vi "Autonomous Independent.vi"() -> ()   [LabVIEW 2020]
doc: "This VI is called when autonomous begins, and will automatically be terminated when autonomous ends. You can carry out timed or sensor driven robot movement independently without needing to return to the caller."
uses:
  <vilib>/Rock Robotics/Network Tables/NT Read String.vi
  <vilib>/Utility/file.llb/Read Delimited Spreadsheet (DBL).vi
  Robot Global Data.vi
  <vilib>/Rock Robotics/WPI/RobotDrive/WPI_RobotDriveArcadeDrive_Standard(NoSaturation).vi
  <vilib>/Rock Robotics/Network Tables/NT Write Numeric Array.vi
panel:
  out "Current Movement, for debugging":T1 {"Y Joystick Value" scale=1.0..-1.0; "X Joystick Value" scale=-1.0..1.0}
  in  "Array of robot movements":T2(array[cluster])=[{"X Joystick Value"=0.39393939393939403, "Y Joystick Value"=0.0, "Delay (sec)"=1.0, "Movement Name"="turn"}, {"X Joystick Value"=-0.3737373737373737, "Y Joystick Value"=0.0, "Delay (sec)"=1.0, "Movement Name"="turn back"}] {"Y Joystick Value" scale=1.0..-1.0; "X Joystick Value" scale=-1.0..1.0}
  # "Be sure to right-click and choose Data Operations>>Make Current Value default if you want to save the array values with the VI"
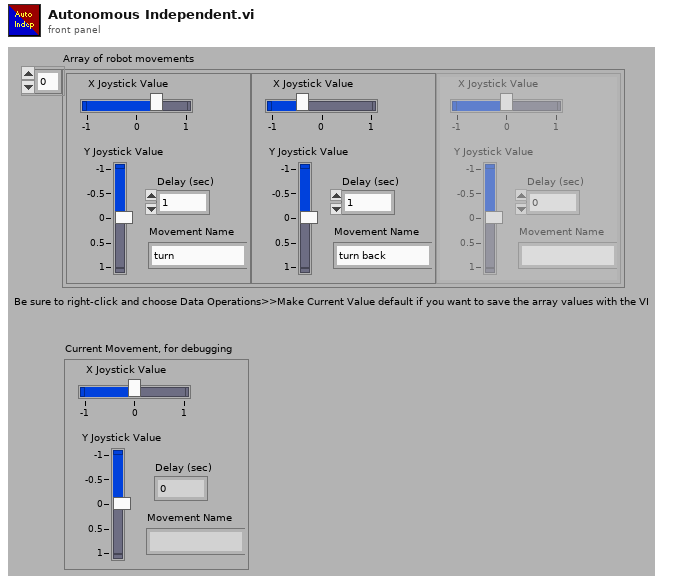
[diagram p1: front panel]
types:
  T1 = cluster{"X Joystick Value":dbl, "Y Joystick Value":dbl, "Delay (sec)":dbl, "Movement Name":string}
  T2 = cluster{"X Joystick Value":dbl, "Y Joystick Value":dbl, "Delay (sec)":dbl, "Movement Name":string}[]
  T3 = typedef "WPI_JoystickDevRef.ctl" = cluster{"Device":T4}
  T4 = typedef "WPI_JoystickDeviceEnum.ctl" = enum16{"USB 0", "USB 1", "USB 2", "USB 3", "USB 4", "USB 5"}
  T5 = typedef "WPI_RobotDriveDevRef.ctl" = cluster{"DevStatus":errorcluster, "Motors[]":T6[], "Square Inputs":bool, "Max Output":dbl}
  T6 = typedef "WPI_MotorControlDeviceRef.ctl" = cluster{"DeviceStatus":errorcluster, "Type":T7, "PWM":cluster{"PWM Channel":T8, "DeadBand":T9}, "CAN":cluster{"Device Number":u8, "SetOutput VI Ref":variant, "GetOutput VI Ref":variant, "Enable VI Ref":variant, "Disable VI Ref":variant, "Data":variant}, "Invert":bool, "DIO PWM":cluster{"PWM \"Enable\" Channel":T8, "DIOChannel":T10, "PWM Rate":dbl}}
  T7 = typedef "WPI_MotorControlType.ctl" = enum16{"PWM", "CAN", "DIO PWM"}
  T8 = typedef "FPGA_DIOPWMChannel.ctl" = enum8{"PWM 0", "PWM 1", "PWM 2", "PWM 3", "PWM 4", "PWM 5", "PWM 6", "PWM 7", "PWM 8", "PWM 9", "PWM MXP 0", "PWM MXP 1", "PWM MXP 2", "PWM MXP 3", "PWM MXP 4", "PWM MXP 5", "PWM MXP 6", "PWM MXP 7", "PWM MXP 8", "PWM MXP 9", "Invalid"}
  T9 = typedef "WPI_PWMDeadband.ctl" = cluster{"Name":string, "maxPositivePwm":i32, "minPositivePwm":i32, "centerPwm":i32, "maxNegativePwm":i32, "minNegativePwm":i32, "angularRange":u16}
  T10 = typedef "FPGA_DIOChannel.ctl" = enum8{"DIO 0", "DIO 1", "DIO 2", "DIO 3", "DIO 4", "DIO 5", "DIO 6", "DIO 7", "DIO 8", "DIO 9", "DIO MXP 0", "DIO MXP 1", "DIO MXP 2", "DIO MXP 3", "DIO MXP 4", "DIO MXP 5", "DIO MXP 6", "DIO MXP 7", "DIO MXP 8", "DIO MXP 9", "DIO MXP 10", "DIO MXP 11", "DIO MXP 12", "DIO MXP 13", "DIO MXP 14", "DIO MXP 15", "SPI Port CS1", "SPI Port CS2", "SPI Port CS3", "SPI Port MISO", "SPI Port MOSI", "Invalid"}
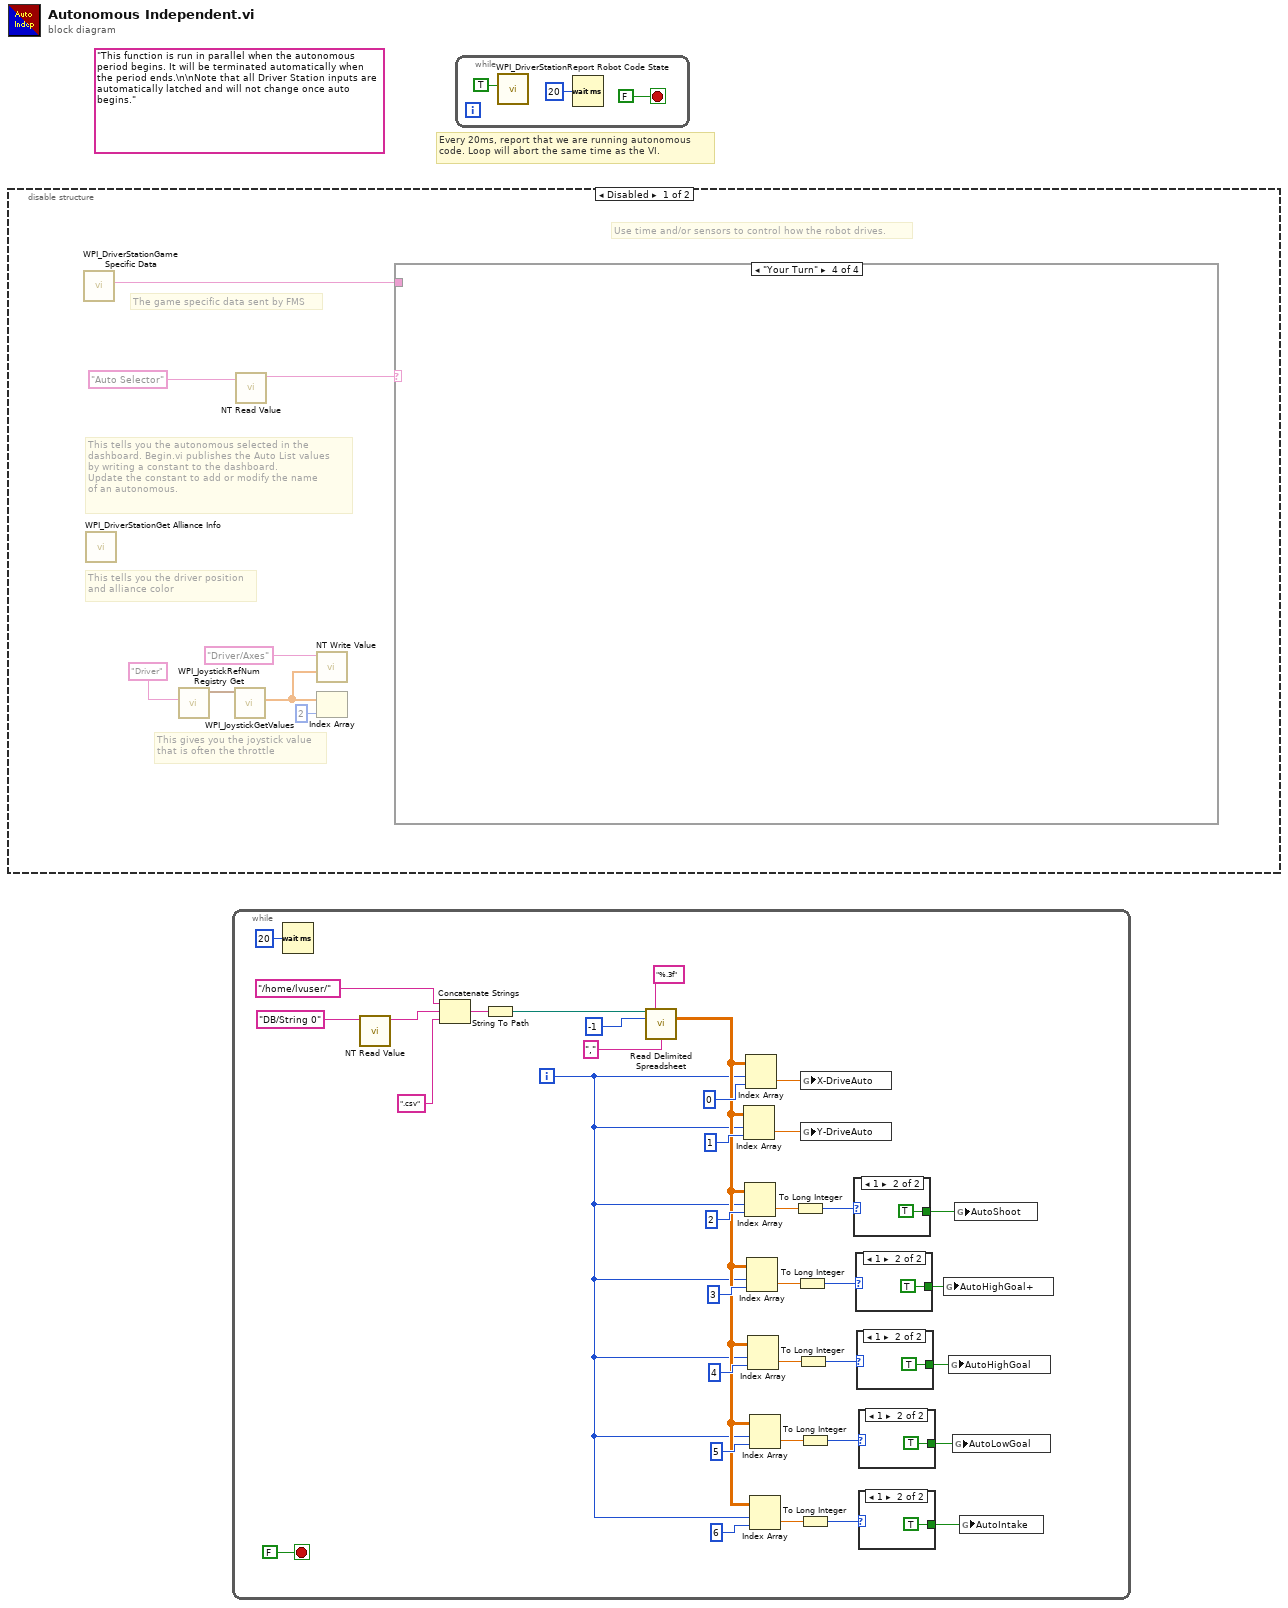
[diagram p0: block diagram]
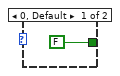
[diagram p2: hidden frame]
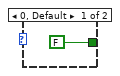
[diagram p3: hidden frame]
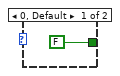
[diagram p4: hidden frame]
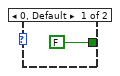
[diagram p5: hidden frame]
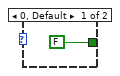
[diagram p6: hidden frame]
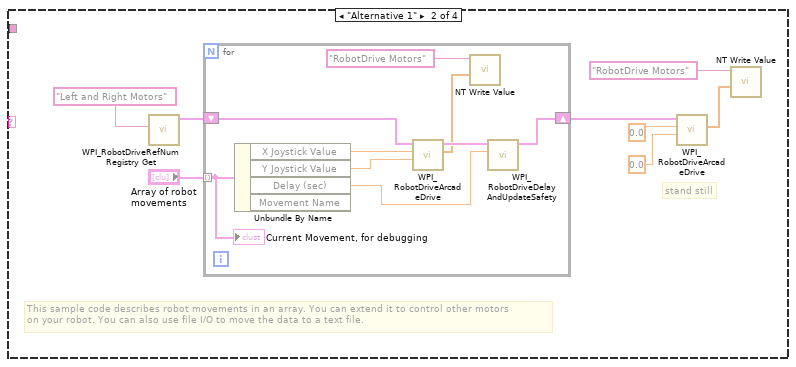
[diagram p8: hidden frame]
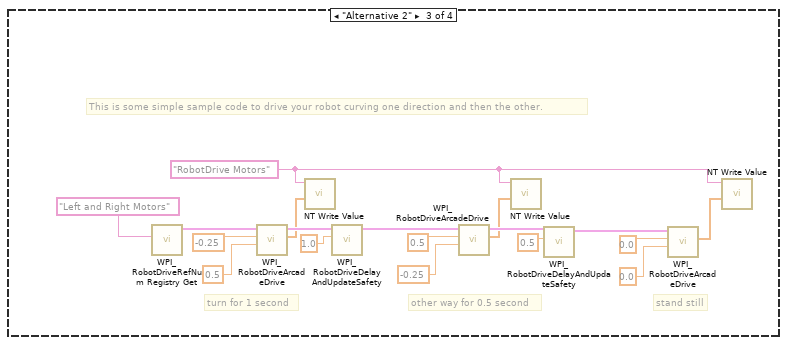
[diagram p9: hidden frame]
diagram:
  (unwired) "This function is run in parallel when the autonomous period begins. It will be terminated automatically when the period ends.\n\nNote that all Driver Station inputs are automatically latched and will not change once auto begins."
  # "Every 20ms, report that we are running autonomous\ncode. Loop will abort the same time as the VI."
  n1 = disable-structure shown="Disabled" {
    frame Disabled {
      # "This gives you the joystick value\nthat is often the throttle"
      # "The game specific data sent by FMS"
      # "This tells you the autonomous selected in the \ndashboard. Begin.vi publishes the Auto List values\nby writing a constant to the dashboard.\nUpdate the constant to add or modify the name\nof an autonomous."
      # "Use time and/or sensors to control how the robot drives."
      # "This tells you the driver position\nand alliance color"
      n2 = call <vilib>:"WPI_DriverStationGame Specific Data.vi"() -> ("Game Specific Data"=w6:string)  [unwired: 11 in]
      n3 = call <vilib>:"WPI_DriverStationGet Alliance Info.vi"() -> ()  [unwired: 12 out]
      n4 = call <vilib>:"WPI_JoystickRefNum Registry Get.vi"("refnum name"="Driver") -> ("JoystickDevRef"=w4:T3)  [unwired: 1 in, 9 out]
      n5 = call <vilib>:"WPI_JoystickGetValues.vi"("JoystickDevRef"=w4) -> ("Axes"=w2:dbl[])  [unwired: 6 in, 4 out]
      n6 = call-poly <vilib>:"NT Read Value.vi"("Name"="Auto Selector") -> ("String"=w7:string)  [unwired: 9 in, 1 out]
      n7 = call-poly <vilib>:"NT Write Value.vi"("Numeric Array"=w2, "Name"="Driver/Axes") -> ()  [unwired: 9 in, 1 out]
      n8 = Index Array(array=w2, index=2) -> ()  [unwired: 1 out]
      n9 = case shown="\"Your Turn\"" w7 {
        tunnel: w6 -> [_ _ _ _]
        frame Default {
          # "You can put your main auto here, or you can right-click on the case and make any\nother frame be the default case."
          # "This is the frame that will execute if no selection is made, or if it is not recognized"
        }
        frame "Alternative 1" {
          # "stand still"
          # "This sample code describes robot movements in an array. You can extend it to control other motors\non your robot. You can also use file I/O to move the data to a text file."
          n10 = call <vilib>:"WPI_RobotDriveRefNum Registry Get.vi"("refnum name"="Left and Right Motors") -> ("RobotDriveDevRef"=w15:T5)  [unwired: 1 in, 9 out]
          n11 = for {
            shift-right: [w23] -> w10
            shift-left: w15 -> [w24]
            tunnel: "Array of robot movements" -> [w19] mode=indexing
            n12 = Unbundle By Name(w19) -> ("X Joystick Value"=w22:dbl, "Y Joystick Value"=w21:dbl, "Delay (sec)"=w20:dbl)  [unwired: 1 out]
            n13 = call-poly <vilib>:"WPI_RobotDriveArcadeDrive.vi"("Y axis value"=w21, "X axis value"=w22, "RobotDriveDevRef"=w24) -> ("Motor Values"=w17:dbl[], "RobotDriveDevRef"=w25:T5)  [unwired: 1 in, 6 out]
            n14 = call-poly <vilib>:"NT Write Value.vi"("Numeric Array"=w17, "Name"="RobotDrive Motors") -> ()  [unwired: 9 in, 1 out]
            n15 = call <vilib>:"WPI_RobotDriveDelayAndUpdateSafety.vi"("Delay (s)"=w20, "RobotDriveDevRef"=w25) -> ("RobotDriveDevRef 2"=w23:T5)  [unwired: 8 in, 1 out]
            "Current Movement, for debugging" <- w19
          }
          n16 = call-poly <vilib>:"WPI_RobotDriveArcadeDrive.vi"("Y axis value"=0.0 ("X axis value"), "X axis value"=0.0, "RobotDriveDevRef"=w10) -> ("Motor Values"=w13:dbl[])  [unwired: 1 in, 7 out]
          n17 = call-poly <vilib>:"NT Write Value.vi"("Numeric Array"=w13, "Name"="RobotDrive Motors") -> ()  [unwired: 9 in, 1 out]
        }
        frame "Alternative 2" {
          w27 = "RobotDrive Motors" ("Name")
          # "This is some simple sample code to drive your robot curving one direction and then the other."
          # "stand still"
          # "other way for 0.5 second"
          # "turn for 1 second"
          n18 = call <vilib>:"WPI_RobotDriveRefNum Registry Get.vi"("refnum name"="Left and Right Motors") -> ("RobotDriveDevRef"=w43:T5)  [unwired: 1 in, 9 out]
          n19 = call-poly <vilib>:"WPI_RobotDriveArcadeDrive.vi"("Y axis value"=0.5 ("X axis value"), "X axis value"=-0.25, "RobotDriveDevRef"=w43) -> ("Motor Values"=w26:dbl[], "RobotDriveDevRef"=w36:T5)  [unwired: 1 in, 6 out]
          n20 = call-poly <vilib>:"NT Write Value.vi"("Numeric Array"=w26, "Name"=w27) -> ()  [unwired: 9 in, 1 out]
          n21 = call <vilib>:"WPI_RobotDriveDelayAndUpdateSafety.vi"("Delay (s)"=1.0, "RobotDriveDevRef"=w36) -> ("RobotDriveDevRef 2"=w37:T5)  [unwired: 8 in, 1 out]
          n22 = call-poly <vilib>:"WPI_RobotDriveArcadeDrive.vi"("Y axis value"=-0.25 ("X axis value"), "X axis value"=0.5, "RobotDriveDevRef"=w37) -> ("Motor Values"=w28:dbl[], "RobotDriveDevRef"=w38:T5)  [unwired: 1 in, 6 out]
          n23 = call-poly <vilib>:"NT Write Value.vi"("Numeric Array"=w28, "Name"=w27) -> ()  [unwired: 9 in, 1 out]
          n24 = call <vilib>:"WPI_RobotDriveDelayAndUpdateSafety.vi"("Delay (s)"=0.5, "RobotDriveDevRef"=w38) -> ("RobotDriveDevRef 2"=w39:T5)  [unwired: 8 in, 1 out]
          n25 = call-poly <vilib>:"WPI_RobotDriveArcadeDrive.vi"("Y axis value"=0.0 ("X axis value"), "X axis value"=0.0, "RobotDriveDevRef"=w39) -> ("Motor Values"=w29:dbl[])  [unwired: 1 in, 7 out]
          n26 = call-poly <vilib>:"NT Write Value.vi"("Numeric Array"=w29, "Name"=w27) -> ()  [unwired: 9 in, 1 out]
        }
        frame "Your Turn" {
        }
      }
    }
    frame Enabled {
    }
  }
  n27 = while {
    i -> [w50]
    stop <- FALSE stop-if-true
    n28 = Wait (ms)(milliseconds to wait=u32 20) -> ()  [unwired: 1 out]
    n29 = call-poly <vilib>:"NT Read Value.vi"("Name"="DB/String 0") -> ("String"=w47:string)  [unwired: 9 in, 1 out]
    n30 = Concatenate Strings("/home/lvuser/", w47, ".csv") -> (w45:string)
    n31 = String To Path(string=w45) -> (path=w44:path)
    n32 = call-poly <vilib>:"Read Delimited Spreadsheet.vi"("file path (dialog if empty)"=w44, "format (%.3f)"="%.3f", "number of rows (all:-1)"=-1, "delimiter (\\t)"="," ("delimiter (\\t)")) -> ("all rows"=w51:dbl[][])  [unwired: 6 in, 5 out]
    n33 = Index Array(array=w51, index (row)=w50, index (col)=1 ("disabled index (col)")) -> (element=w72:dbl)
    n34 = Index Array(array=w51, index (row)=w50, index (col)=2 ("disabled index (col)")) -> (element=w70:dbl)
    n35 = Index Array(array=w51, index (row)=w50, index (col)=0 ("disabled index (col)")) -> (element=w73:dbl)
    n36 = Index Array(array=w51, index (row)=w50, index (col)=3 ("disabled index (col)")) -> (element=w66:dbl)
    n37 = Index Array(array=w51, index (row)=w50, index (col)=4 ("disabled index (col)")) -> (element=w62:dbl)
    n38 = Index Array(array=w51, index (row)=w50, index (col)=5 ("disabled index (col)")) -> (element=w58:dbl)
    n39 = Index Array(array=w51, index (row)=w50, index (col)=6 ("disabled index (col)")) -> (element=w54:dbl)
    n40 = To Long Integer(number=w70) -> (32bit integer=w68:i32)
    n41 = To Long Integer(number=w66) -> (32bit integer=w64:i32)
    n42 = To Long Integer(number=w62) -> (32bit integer=w60:i32)
    n43 = To Long Integer(number=w58) -> (32bit integer=w56:i32)
    n44 = To Long Integer(number=w54) -> (32bit integer=w52:i32)
    n45 = global write "Robot Global Data.vi" "X-DriveAuto"(w73) -> ()
    n46 = global write "Robot Global Data.vi" "Y-DriveAuto"(w72) -> ()
    n47 = case shown="1" w68 {
      tunnel: [FALSE TRUE] -> w69
      frame 0, Default {
      }
      frame 1 {
      }
    }
    n48 = case shown="1" w64 {
      tunnel: [FALSE TRUE] -> w65
      frame 0, Default {
      }
      frame 1 {
      }
    }
    n49 = case shown="1" w60 {
      tunnel: [FALSE TRUE] -> w61
      frame 0, Default {
      }
      frame 1 {
      }
    }
    n50 = case shown="1" w56 {
      tunnel: [FALSE TRUE] -> w57
      frame 0, Default {
      }
      frame 1 {
      }
    }
    n51 = case shown="1" w52 {
      tunnel: [FALSE TRUE] -> w53
      frame 0, Default {
      }
      frame 1 {
      }
    }
    n52 = global write "Robot Global Data.vi" "AutoHighGoal+"(w65) -> ()
    n53 = global write "Robot Global Data.vi" "AutoHighGoal"(w61) -> ()
    n54 = global write "Robot Global Data.vi" "AutoLowGoal"(w57) -> ()
    n55 = global write "Robot Global Data.vi" "AutoShoot"(w69) -> ()
    n56 = global write "Robot Global Data.vi" "AutoIntake"(w53) -> ()
  }
  n57 = while {
    stop <- FALSE stop-if-true
    n58 = call <vilib>:"WPI_DriverStationReport Robot Code State.vi"("Autonomous"=TRUE) -> ()  [unwired: 10 in, 1 out]
    n59 = Wait (ms)(milliseconds to wait=u32 20) -> ()  [unwired: 1 out]
  }
